vi "GetChangedEdges.vi"(8 "error in (no error)":errorcluster, 10 "Apply Updates (F)":bool, 11 "OccupancyGridWorldMap in":refnum<class "NI_Robotics_OccupancyGridWorldMap.lvclass">) -> (0 "error out":errorcluster, 2 "Changed Edges":T1[](array[typedef]), 3 "OccupancyGridWorldMap out":refnum<class "NI_Robotics_OccupancyGridWorldMap.lvclass">)   [LabVIEW 2017, in "NI_Robotics_OccupancyGridWorldMap.lvclass"]
uses:
  <vilib>/robotics/Navigation/shared/WorldMap/OccupancyGridWorldMap/NI_Robotics_OccupancyGridWorldMap.lvclass
  <vilib>/robotics/Navigation/shared/WorldMap/World Map Edge.ctl
  <vilib>/robotics/Navigation/shared/MapNode/AbstractMapNode/NI_Robotics_AbstractMapNode.lvclass
  <vilib>/robotics/Navigation/shared/WorldMap/OccupancyGridWorldMap/NI_Robotics_OccupancyGridWorldMap.lvclass/NI_Robotics_OccupancyGridWorldMap.ctl
  <vilib>/robotics/Navigation/shared/MapNode/OccupancyGridNode/NI_Robotics_OccupancyGridMapNode.lvclass
  c:/Program Files (x86)/National Instruments/LabVIEW 2017/vi.lib/robotics/Navigation/shared/MapNode/AbstractMapNode/NI_Robotics_AbstractMapNode.lvclass
  <vilib>/robotics/Navigation/shared/WorldMap/AbstractWorldMap/NI_Robotics_AbstractWorldMap.lvclass
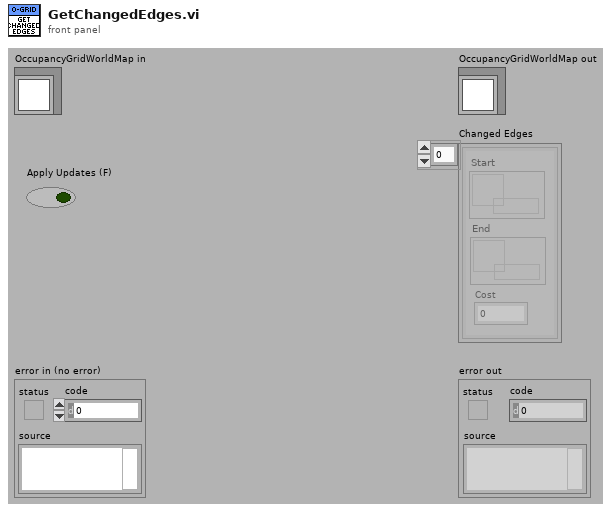
[diagram p1: front panel]
types:
  T1 = typedef "NI_Robotics_AbstractWorldMap.lvclass/World Map Edge.ctl" = cluster{"Start":refnum<data-value>, "End":refnum<data-value>, "Cost":dbl}
  T2 = cluster{"NodeReference 2":refnum<data-value>, "NodeReference 2":refnum<data-value>, "Cost":dbl}[]
  T3 = cluster{"NodeReference 2":refnum<data-value>, "NodeReference 2":refnum<data-value>, "Cost":dbl}
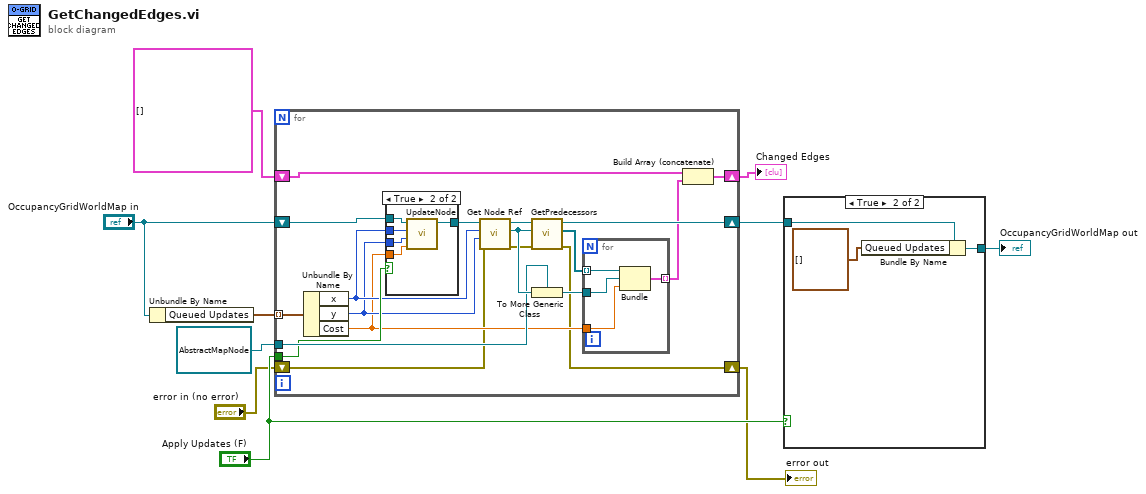
[diagram p0: block diagram]
diagram:
  n1 = Unbundle By Name("OccupancyGridWorldMap in") -> ("Queued Updates"=w10:cluster{"x":i32, "y":i32, "Cost":dbl}[])
  n2 = for {
    tunnel: w10 -> [w29] mode=indexing
    shift-right: [w27] -> w4
    shift-left: "OccupancyGridWorldMap in" -> [w15]
    shift-right: [w22] -> w6
    shift-left: T2 [] -> [w17]
    tunnel: refnum<data-value> refnum ("NodeReference 2") -> [w24]
    tunnel: "Apply Updates (F)" -> [w21]
    shift-right: [w11] -> w1
    shift-left: "error in (no error)" -> [w12]
    n3 = Unbundle By Name(w29) -> ("x"=w20:i32, "y"=w19:i32, "Cost"=w18:dbl)
    n4 = case shown="True" w21 {
      tunnel: w20 -> [_ w35]
      tunnel: w15 -> [w30 w34]
      tunnel: w19 -> [_ w33]
      tunnel: w18 -> [_ w32]
      tunnel: [w30 w31] -> w14
      frame False {
      }
      frame True {
        n5 = call-dynamic "UpdateNode.vi"("Cost"=w32, "y"=w33, "x"=w35, "OccupancyGridWorldMap in"=w34) -> ("OccupancyGridWorldMap out"=w31:refnum<class "NI_Robotics_OccupancyGridWorldMap.lvclass">)  [unwired: 7 in]
      }
    }
    n6 = call <vilib>:"Get Node Ref.vi"("error in (no error)"=w12, "y"=w19, "x"=w20, "OccupancyGridWorldMap in"=w14) -> ("error out"=w13:errorcluster, "element"=w25:refnum<data-value>, "OccupancyGridWorldMap out"=w28:refnum<class "NI_Robotics_OccupancyGridWorldMap.lvclass">)  [unwired: 4 in, 1 out]
    n7 = call-dynamic "GetPredecessors.vi"("error in (no error)"=w13, "NodeReference"=w25, "WorldMap in"=w28) -> ("error out"=w11:errorcluster, "Predecessors"=w26:refnum<data-value>[], "WorldMap out"=w27:refnum<class "NI_Robotics_OccupancyGridWorldMap.lvclass">)  [unwired: 5 in, 1 out]
    n8 = To More Generic Class(target class=w24, reference=w25) -> (generic class reference=w23:refnum<data-value>)
    n9 = for {
      tunnel: w26 -> [w38] mode=indexing
      tunnel: w18 -> [w37]
      tunnel: w23 -> [w39]
      tunnel: [w36] -> w16 mode=indexing
      n10 = Bundle("NodeReference 2"=w38, "NodeReference 2"=w39, "Cost"=w37) -> (w36:T3)  [unwired: 1 in]
    }
    n11 = Build Array (concatenate)(w17, w16) -> (w22:T2)
  }
  "error out" <- w1
  "Changed Edges" <- w6
  n12 = case shown="True" "Apply Updates (F)" {
    tunnel: w4 -> [w40 w43]
    tunnel: [w40 w41] -> w3
    frame False {
    }
    frame True {
      n13 = Bundle By Name(cluster=w43, "Queued Updates"=cluster{"x":i32, "y":i32, "Cost":dbl}[] []) -> (w41:refnum<class "NI_Robotics_OccupancyGridWorldMap.lvclass">)
    }
  }
  "OccupancyGridWorldMap out" <- w3
